vi "Add VI to Virtual Folder.vi"(7 "Virtual Folder":refnum<vi>, 8 "error in":errorcluster, 10 "VI Name":string, 11 "Path to VI":path) -> (0 "error out":errorcluster, 3 "Path to VI":path)   [LabVIEW 2014, in "Initialization and IO Node Scripting.lvlib"]
uses:
  Initialization and IO Node Scripting.lvlib
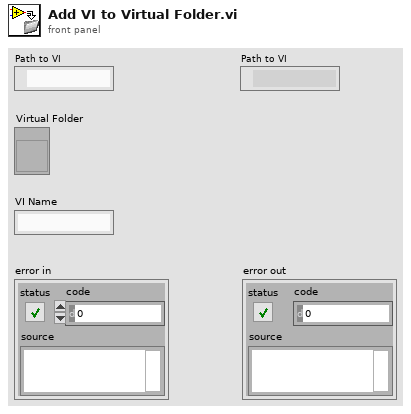
[diagram p1: front panel]
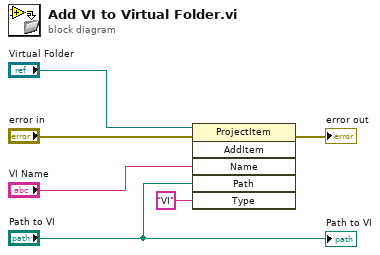
[diagram p0: block diagram]
diagram:
  n1 = invoke class="ProjectItem" method="AddItem"(reference="Virtual Folder", error in="error in", "Name"="VI Name", "Path"="Path to VI", "Type"="VI") -> (error out=→"error out":errorcluster)  [unwired: 1 in, 5 out]
  "Path to VI" <- "Path to VI"
